vi "E441X_PM_Build_Measure_Command.vi"(0 "VISA session":refnum<visa-resource-name>, 1 "Measurement (1)":i32=1 step=1, 2 "Command":string, 3 "Question (F: No Question)":bool, 5 "Measuring Function (0: Single)":i32(ring) items=["Single", "Single Relative", "Difference", "Difference Relative", "Ratio", "Ratio Relative"], 7 "Sensor 1 (0: Channel A)":i32(ring) items=["Channel A", "Channel B"], 9 "Sensor 2 (0: Channel A)":i32(ring) items=["Channel A", "Channel B"], 11 "error in (no error)":errorcluster {"code" format="%.0x"}, 12 "Resolution (3)":i32=3 step=1, 13 "Expected Value (0.00)":dbl format="%.2f", 14 "Expected Value (F: Off)":bool) -> (4 "dup VISA session":refnum<visa-resource-name>, 8 "Output Command":string, 15 "error out":errorcluster {"code" format="%.0x"})   [LabVIEW 2015]
doc: "This VI formats the measurement command."
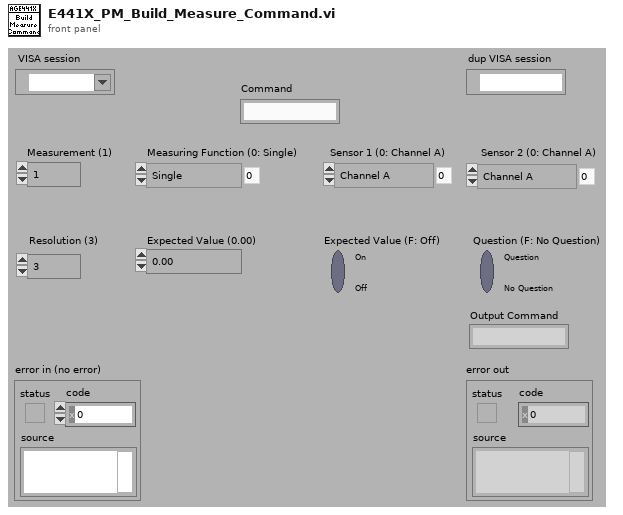
[diagram p1: front panel]
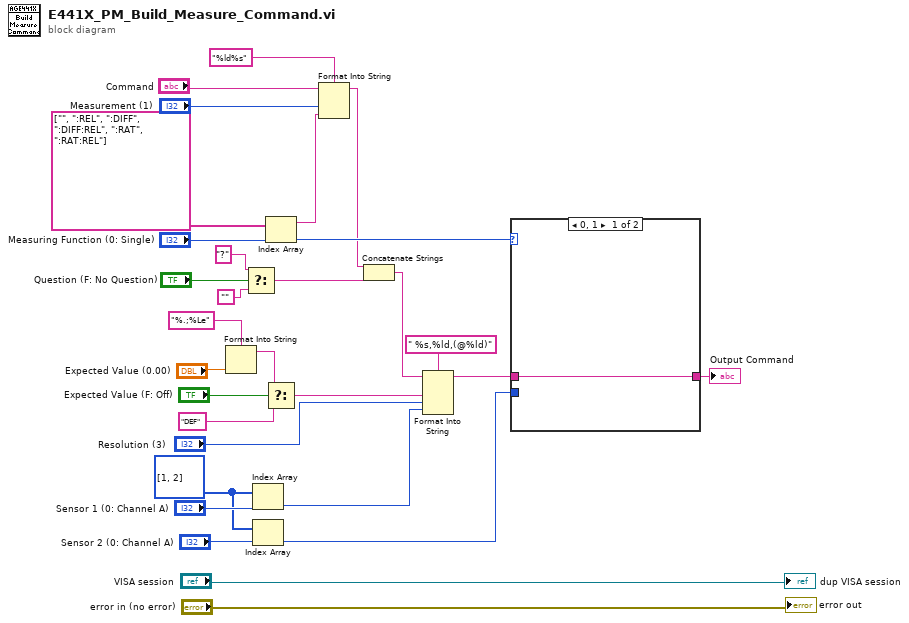
[diagram p0: block diagram]
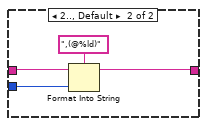
[diagram p2: hidden frame]
diagram:
  w6 = i32[] [1, 2]
  n1 = Format Into String(format string="%.;%Le", "Expected Value (0.00)") -> (resulting string=w16:string)  [unwired: 2 in, 1 out]
  n2 = Select(t="?" ("format string"), s="Question (F: No Question)", f="") -> (s? t:f=w20:string)
  n3 = Index Array(array=w6, index="Sensor 1 (0: Channel A)") -> (element=w8:i32)
  n4 = Index Array(array=w6, index="Sensor 2 (0: Channel A)") -> (element=w4:i32)
  n5 = Index Array(array=string[] ["", ":REL", ":DIFF", ":DIFF:REL", ":RAT", ":RAT:REL"], index="Measuring Function (0: Single)") -> (element=w24:string)
  n6 = Select(t=w16, s="Expected Value (F: Off)", f="DEF") -> (s? t:f=w11:string)
  n7 = Format Into String(format string="%ld%s", initial string="Command", "Measurement (1)", w24) -> (resulting string=w21:string)  [unwired: 1 in, 1 out]
  n8 = Concatenate Strings(w21, w20) -> (w13:string)
  n9 = Format Into String(format string=" %s,%ld,(@%ld)", initial string=w13, w11, "Resolution (3)", w8) -> (resulting string=w7:string)  [unwired: 1 in, 1 out]
  n10 = case shown="0, 1" "Measuring Function (0: Single)" {
    tunnel: [w30 w32] -> w3
    tunnel: w7 -> [w30 w34]
    tunnel: w4 -> [_ w31]
    frame 0, 1 {
    }
    frame 2.., Default {
      n11 = Format Into String(format string=",(@%ld)", initial string=w34, w31) -> (resulting string=w32:string)  [unwired: 1 in, 1 out]
    }
  }
  "Output Command" <- w3
  "error out" <- "error in (no error)"
  "dup VISA session" <- "VISA session"
